vi "Round_DBL_to_String.vi"(1 "Double":dbl, 2 "abs?":bool) -> (0 "String":string)   [LabVIEW 2018]
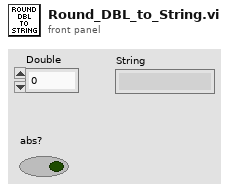
[diagram p1: front panel]
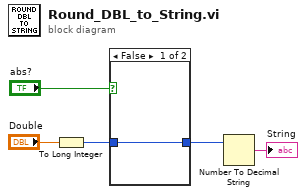
[diagram p0: block diagram]
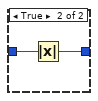
[diagram p2: hidden frame]
diagram:
  n1 = To Long Integer(number="Double") -> (32bit integer=w5:i32)
  n2 = case shown="False" "abs?" {
    tunnel: w5 -> [w6 w8]
    tunnel: [w6 w7] -> w4
    frame False {
    }
    frame True {
      n3 = Absolute Value(x=w8) -> (abs(x)=w7:i32)
    }
  }
  n4 = Number To Decimal String(number=w4) -> (decimal integer string=→"String":string)  [unwired: 1 in]
